vi "main.vi"() -> ()   [LabVIEW 2026]
uses:
  <vilib>/httpClient/LabVIEWHTTPClient.lvlib
panel:
  in  "Fetch Data":bool
  in  "End Date":timestamp
  in  "Start Date":timestamp
  in  "Stop Execution":bool
  out "Air Quality Graph":i32[](graph)
  in  "API Key Token":string
  in  "Parameter Type":u16(ring) items=["PM10"=35875, "PM2.5"=35870, "NO2"=35906]
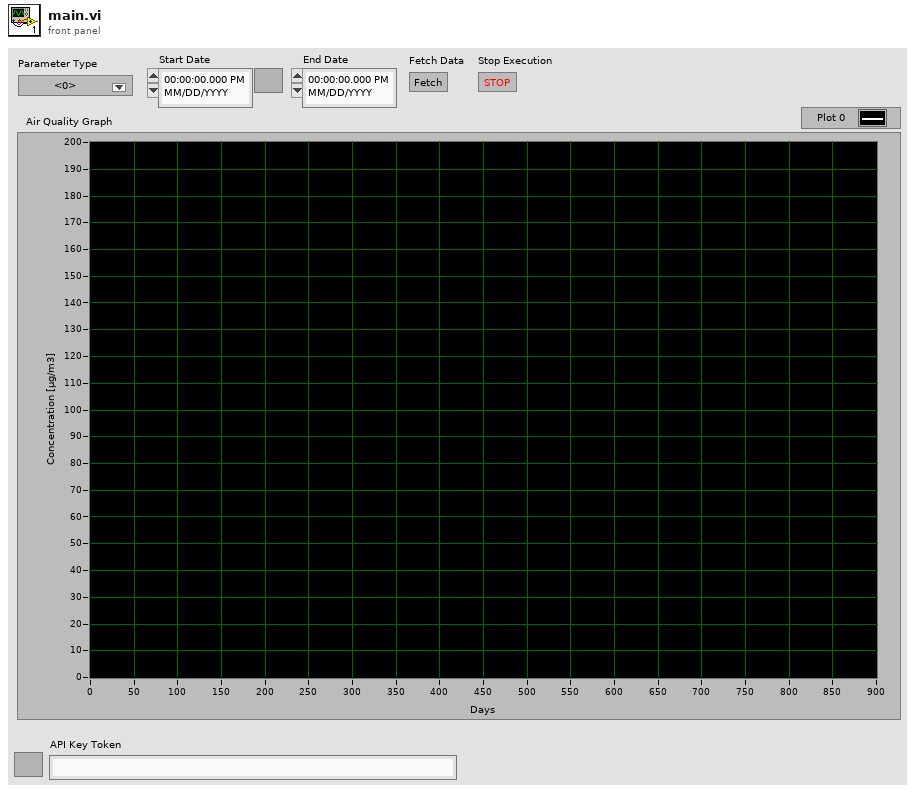
[diagram p1: front panel]
types:
  T1 = cluster{"results":cluster{"value":i32, "period":cluster{"datetimeFrom":cluster{"utc":string}}}[]}
  T2 = typedef "LabVIEWHTTPClient.lvlib/ClientHandle.ctl" = refnum<k1>
  T3 = cluster{"value":i32, "period":cluster{"datetimeFrom":cluster{"utc":string}}}[]
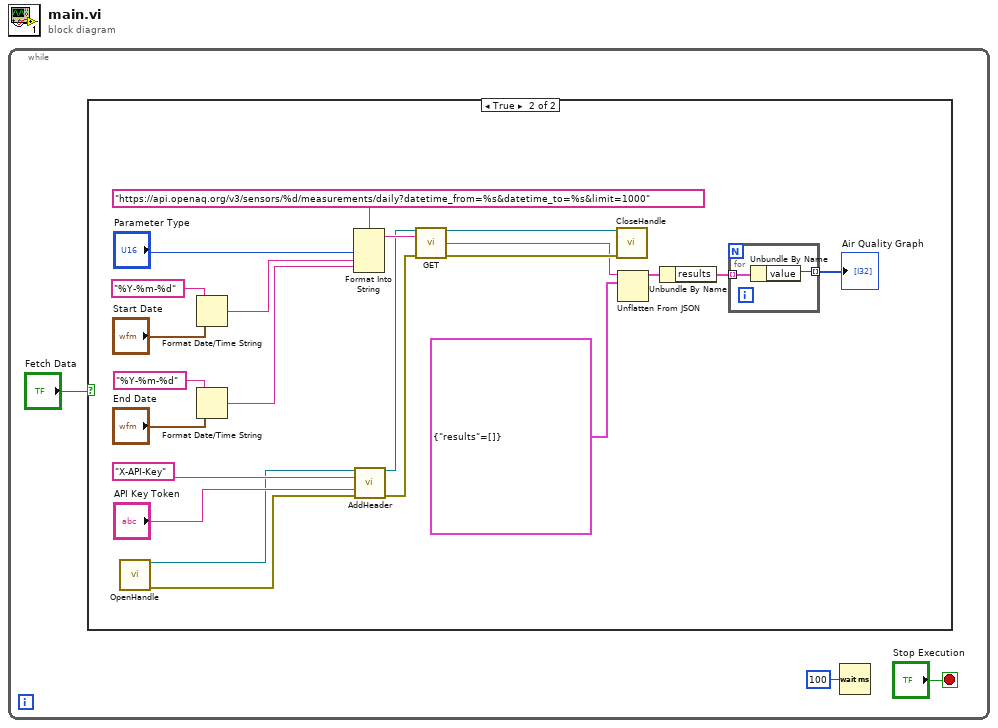
[diagram p0: block diagram]
diagram:
  n1 = while {
    stop <- "Stop Execution" stop-if-true
    n2 = case shown="True" "Fetch Data" {
      frame False {
      }
      frame True {
        n3 = call <vilib>:"OpenHandle.vi"() -> ("client handle out"=w14:T2, "error out"=w13:errorcluster)  [unwired: 14 in]
        n4 = Format Date/Time String(time format string (%c)="%Y-%m-%d", seconds (now)="Start Date") -> (date/time string=w19:string)  [unwired: 1 in]
        n5 = Format Date/Time String(time format string (%c)="%Y-%m-%d", seconds (now)="End Date") -> (date/time string=w18:string)  [unwired: 1 in]
        n6 = Format Into String(format string="https://api.openaq.org/v3/sensors/%d/measurements/daily?datetime_from=%s&datetime_to=%s&limit=1000", "Parameter Type", w19, w18) -> (resulting string=w15:string)  [unwired: 2 in, 1 out]
        n7 = call <vilib>:"AddHeader.vi"("client handle"=w14, "header"="X-API-Key", "value"="API Key Token", "error in (no error)"=w13) -> ("client handle out"=w12:T2, "error out"=w11:errorcluster)  [unwired: 10 in]
        n8 = call <vilib>:"GET.vi"("client handle"=w12, "url"=w15, "error in (no error)"=w11) -> ("client handle out"=w10:T2, "body"=w8:string, "error out"=w9:errorcluster)  [unwired: 9 in, 1 out]
        n9 = call <vilib>:"CloseHandle.vi"("client handle"=w10, "error in (no error)"=w9) -> ()  [unwired: 13 in, 1 out]
        n10 = Unflatten From JSON(JSON string=w8, type and defaults=T1 {"results"=[]}) -> (value=w6:T1)  [unwired: 5 in, 1 out]
        n11 = Unbundle By Name(w6) -> ("results"=w5:T3)
        n12 = for {
          tunnel: w5 -> [w27] mode=indexing
          tunnel: [w26] -> w4 mode=indexing
          n13 = Unbundle By Name(w27) -> ("value"=w26:i32)
        }
        "Air Quality Graph" <- w4
      }
    }
    n14 = Wait (ms)(milliseconds to wait=u32 100) -> ()  [unwired: 1 out]
  }
